vi "Rasnik_20190107.vi"() -> ()   [LabVIEW 2015]
uses:
  GlobalPath.vi
  GlobalData.vi
  <vilib>/Utility/file.llb/Read Delimited Spreadsheet (string).vi
  <vilib>/Utility/file.llb/Write Delimited Spreadsheet (DBL).vi
panel:
  in  "Done?":bool
  in  "Stage":string
  in  "driver off":bool caption="Disconnect the driver from the power supply"
  out "text":string
  out "PanelName":string
  out "appended path":path
  out "Y Diff10":dbl format="%.2f"
  out "Y Diff9":dbl format="%.2f"
  out "Y Diff8":dbl format="%.2f"
  out "Y Diff7":dbl format="%.2f"
  out "Y Diff6":dbl format="%.2f"
  out "Y Diff5":dbl format="%.2f"
  out "Y Diff4":dbl format="%.2f"
  out "Y Diff3":dbl format="%.2f"
  out "Y Diff2":dbl format="%.2f"
  out "Y Diff1":dbl format="%.2f"
  out "X Diff10":dbl format="%.2f"
  out "X Diff9":dbl
  out "X Diff8":dbl format="%.2f"
  out "X Diff7":dbl format="%.2f"
  out "X Diff6":dbl format="%.2f"
  out "X Diff5":dbl format="%.2f"
  out "X Diff4":dbl format="%.2f"
  out "X Diff3":dbl format="%.2f"
  out "X Diff2":dbl format="%.2f"
  out "X Diff1":dbl format="%.2f"
  out "all rows":string[][](array[string])
  out "Y D10":dbl format="%.2f"
  out "Y D9":dbl format="%.2f"
  out "Y D8":dbl format="%.2f"
  out "Y D7":dbl format="%.2f"
  out "Y D6":dbl format="%.2f"
  out "Y D5":dbl format="%.2f"
  out "Y D4":dbl format="%.2f"
  out "Y D3":dbl format="%.2f"
  out "Y D2":dbl format="%.2f"
  out "Y D1":dbl format="%.2f"
  out "X D10":dbl format="%.2f"
  out "X D9":dbl format="%.2f"
  out "X D8":dbl format="%.2f"
  out "X D7":dbl format="%.2f"
  out "X D6":dbl format="%.2f"
  out "X D5":dbl format="%.2f"
  out "X D4":dbl format="%.2f"
  out "X D3":dbl format="%.2f"
  out "X D2":dbl format="%.2f"
  out "X D1":dbl format="%.2f"
  out "y 6":string
  out "y 10":string
  out "y 9":string
  out "y 8":string
  out "y 7":string
  out "y 5":string
  out "y 4":string
  out "y 3":string
  out "y 2":string
  out "y 1":string
  out "x 6":string
  out "x 10":string
  out "x 9":string
  out "x 8":string
  out "x 7":string
  out "x 5":string
  out "x 4":string
  out "x 3":string
  out "x 2":string
  out "x 1":string
  out "output file":path=path "/home/atlas/Micromegas/ProdData/C_CCD/CalcDiscr.txt"
  out "Script":path
  out "Filename selected":path
  out "standard output":string
  in  "Done?":bool
  out "Latest file:":path
  in  "Open Program":bool
  in  "c-ccd 3":bool caption="Setup the electronics for the C-CCD reading:\n- make sure the ethernet cables are connected on the minimal heads\n- check that the cables connecting the driver with the muxs are plugged in\n- CONNECT the driver to the power supply and check that it is connected to the LAN\nIf the measurements show -1 in all c-ccds:\nUNPLUG the driver, WAIT a couple of seconds and REPLUG it"
  in  "c-ccd":bool caption="Read the data file"
  # "Rasmask reading from PCBs on stiffback/table"
  # "Type \"Table\" or \"Stiffback\" for the C-CCDs you want to use:"
  # "Run the C-CCD reading program \n(the 10 Rasmasks are automatically read and the data saved)"
  # "Data file reading"
  # "The most recent data file created by the C-CCD program will be opened.\nOnce the \"read data file\" is clicked, the raw data and displacement should appear on the PCB schematics on the bottom."
  # "Raw Data (mm):"
  # "Calibrated position (mm):"
  # "Difference (wrt Reference reading) (um):"
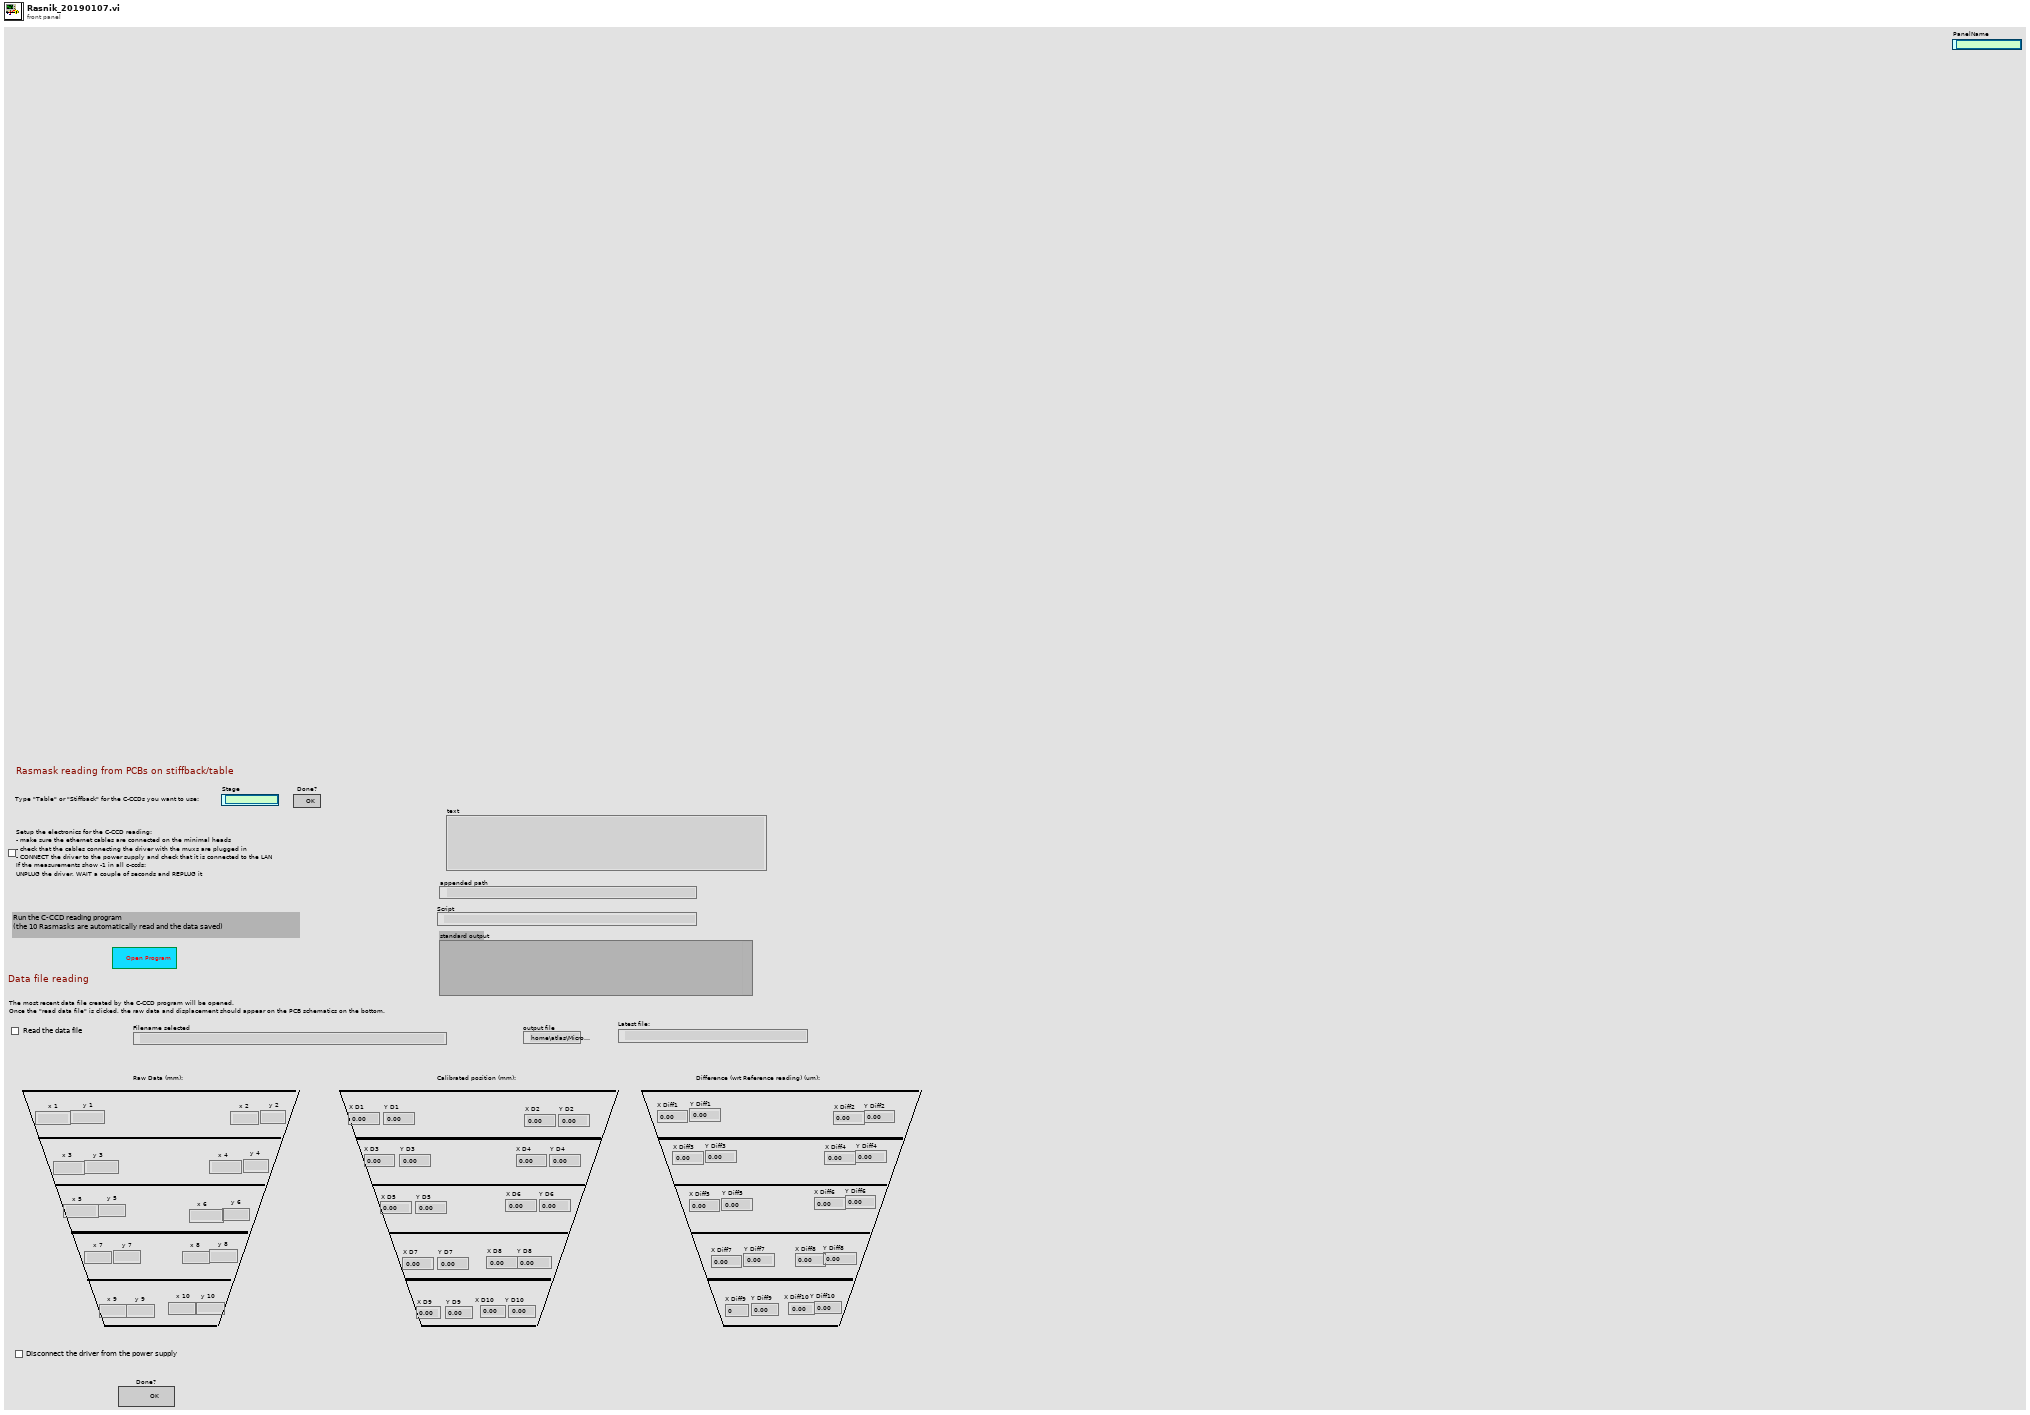
[diagram p1: front panel]
types:
  T1 = enum16{"open", "replace", "create", "open or create", "replace or create", "replace or create with confirmation"}
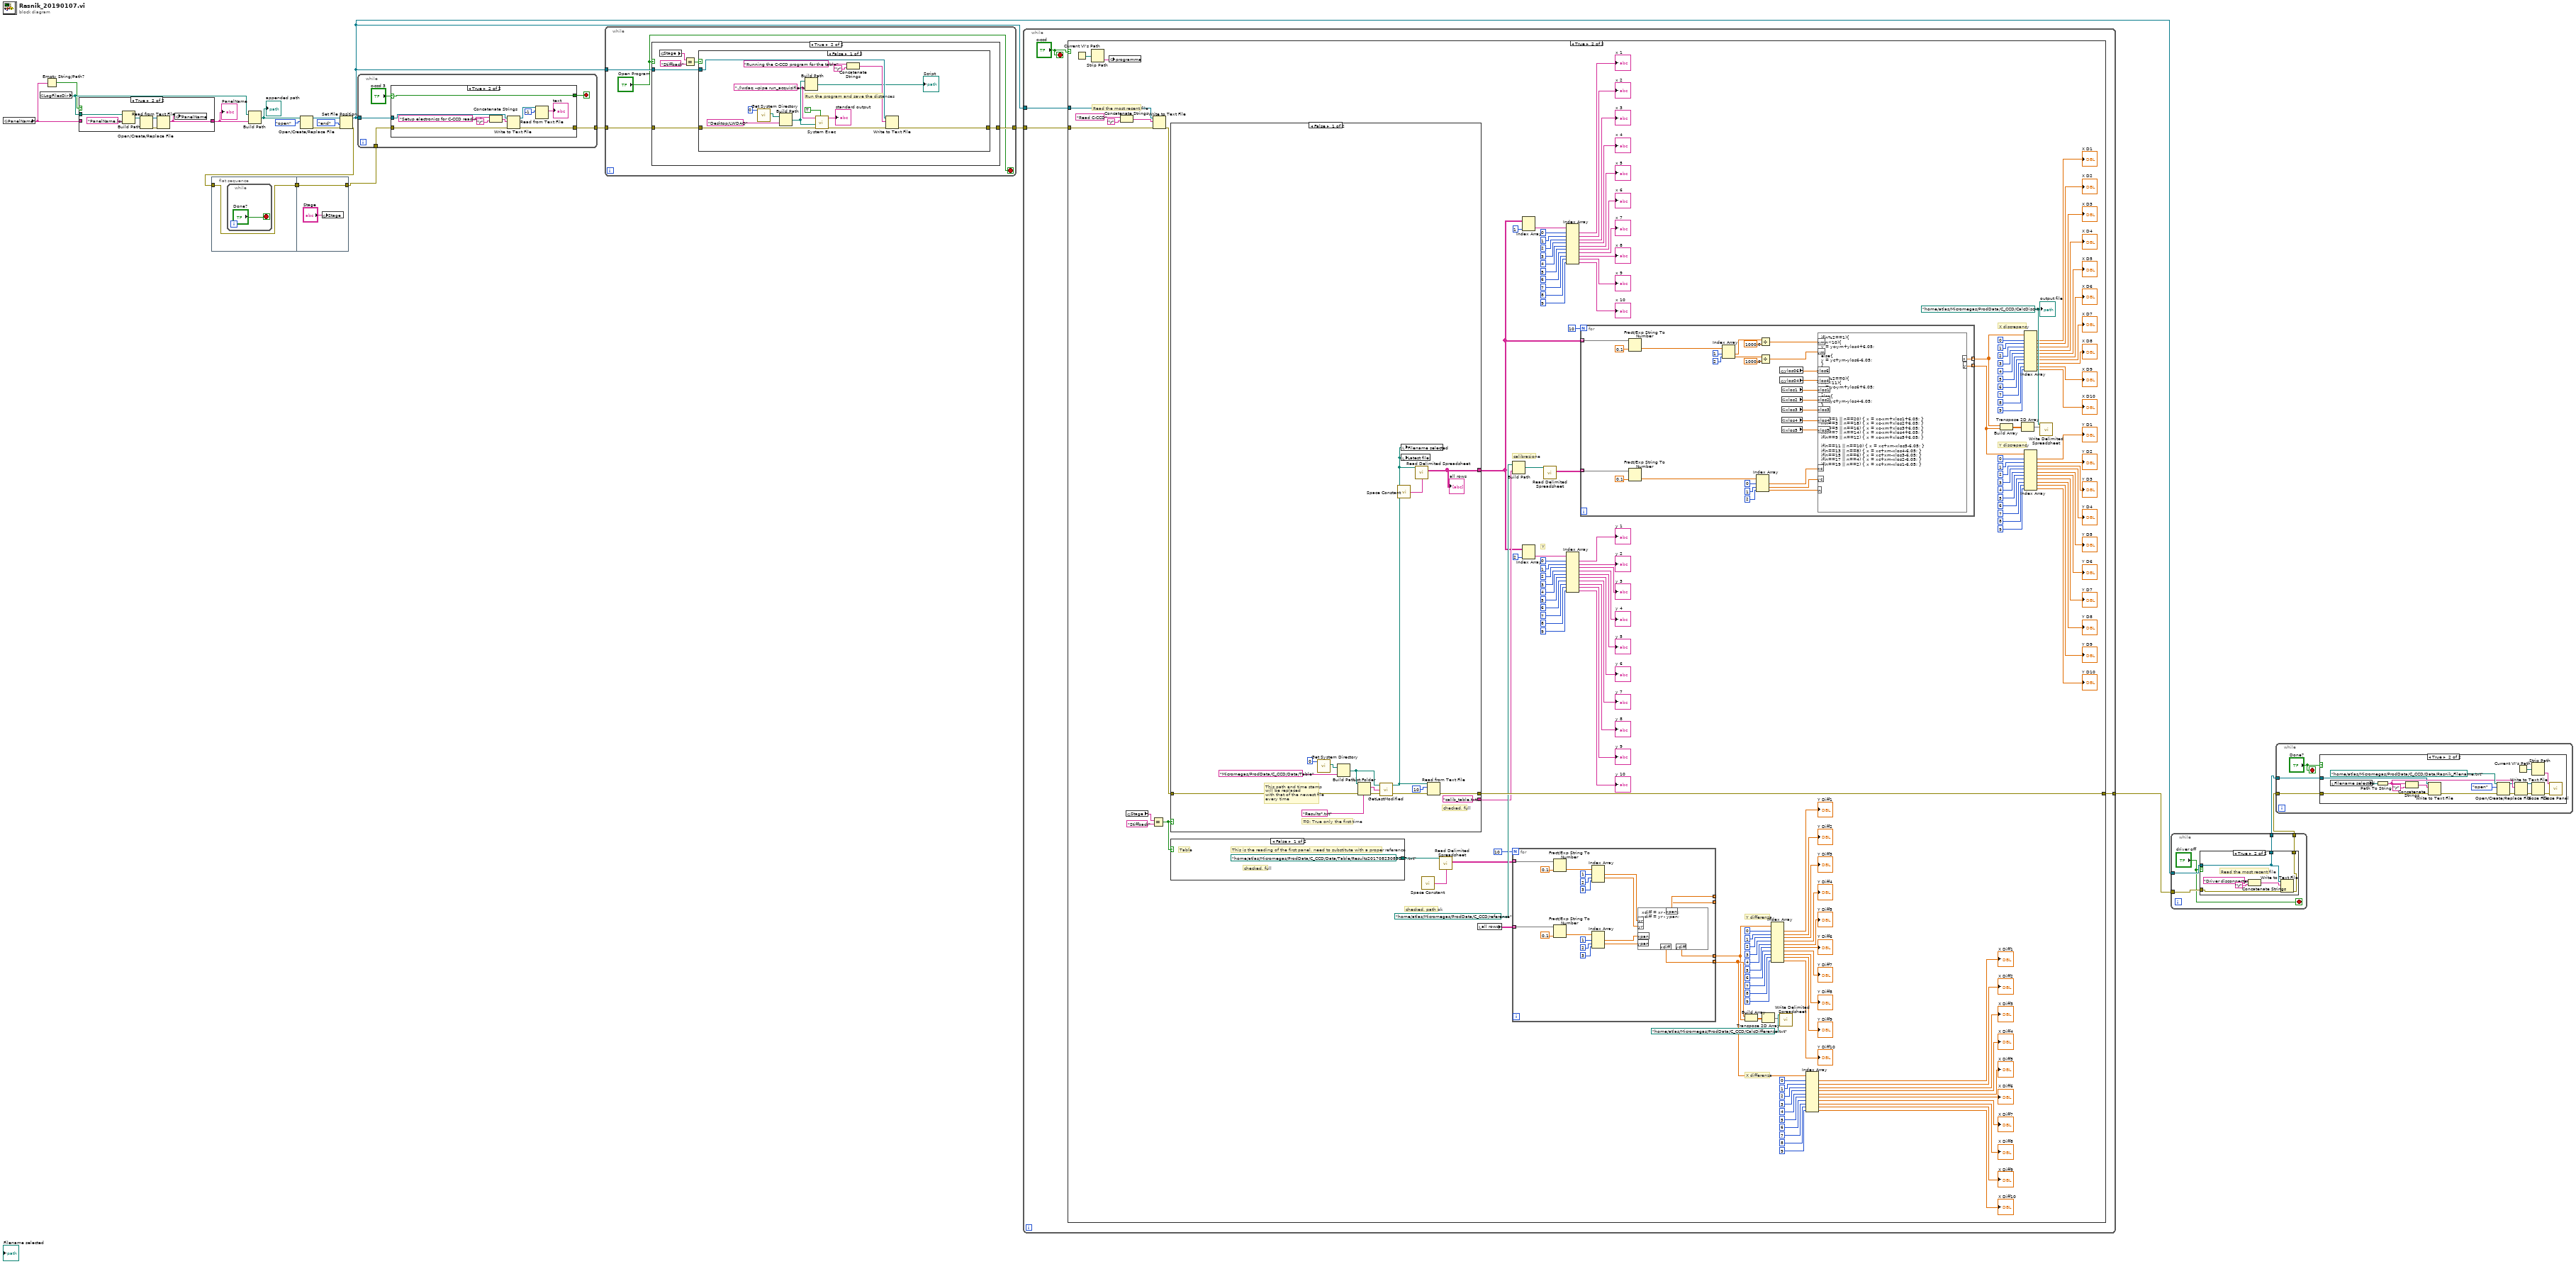
[diagram p0: block diagram]
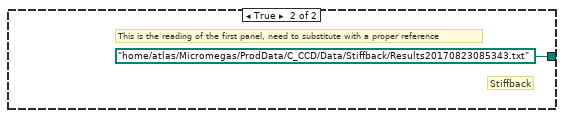
[diagram p5: hidden frame]
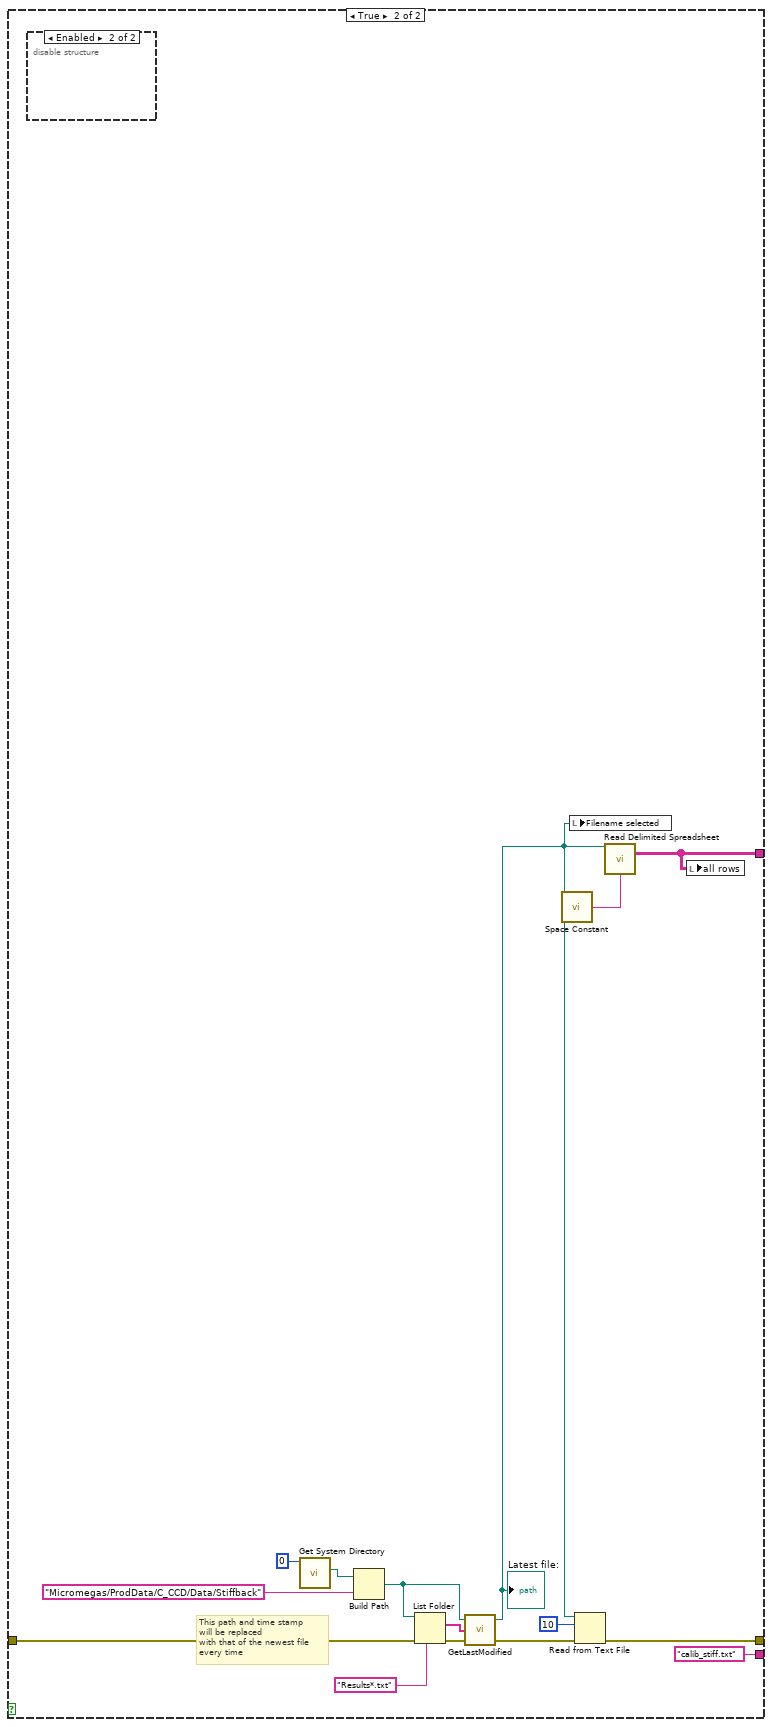
[diagram p6: hidden frame]
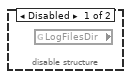
[diagram p7: hidden frame]
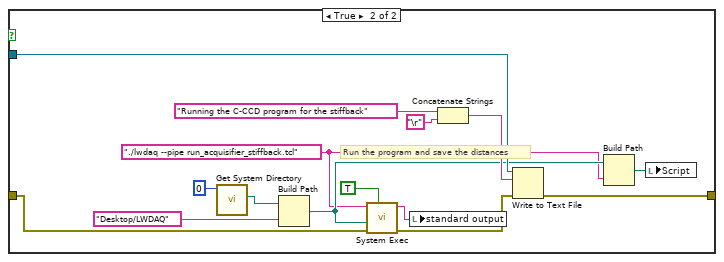
[diagram p10: hidden frame]
diagram:
  n1 = global read "GlobalData.vi" "PanelName"() -> (w14:string)
  n2 = global read "GlobalPath.vi" "LogFilesDir"() -> (w15:path)
  n3 = Empty String/Path?(string/path=w14) -> (empty?=w13:bool)
  n4 = case shown="True" w13 {
    tunnel: w15 -> [_ w25]
    tunnel: [w19 w20] -> w16
    tunnel: w14 -> [w19 _]
    frame False {
    }
    frame True {
      n5 = Build Path(base path=w25, name or relative path="PanelName.log") -> (appended path=w24:path)
      n6 = Open/Create/Replace File(file path (use dialog)=w24) -> (refnum out=w21:refnum<file>, error out=w22:errorcluster)  [unwired: 5 in, 1 out]
      n7 = Read from Text File(file (use dialog)=w21, error in=w22) -> (text=w20:string)  [unwired: 2 in, 3 out]
      n8 = global write "GlobalData.vi" "PanelName"(w20) -> ()
    }
  }
  "PanelName" <- w16
  n9 = flat-sequence {
    tunnel: w3 -> [w26]
    tunnel: [w26] -> w2
    tunnel: [w28] -> w1
    tunnel: w2 -> [w28]
    frame #0 {
      n10 = while {
        stop <- "Done?" stop-if-true
      }
    }
    frame #1 {
      n11 = global write "GlobalData.vi" "Stage"("Stage") -> ()
    }
  }
  n12 = Build Path(base path=w15, name or relative path=w16) -> (appended path=w8:path)
  "appended path" <- w8
  n13 = Open/Create/Replace File(file path (use dialog)=w8, operation (0:open)=T1."open") -> (refnum out=w11:refnum<file>, error out=w12:errorcluster)  [unwired: 4 in, 1 out]
  n14 = Set File Position(refnum=w11, from (0:start)=enum16{"start", "end", "current"}."end", error in=w12) -> (refnum out=w7:refnum<file>, error out=w3:errorcluster)  [unwired: 1 in]
  n15 = while {
    tunnel: w7 -> [w33]
    tunnel: [w31] -> w17
    tunnel: w1 -> [w30]
    stop <- w32 stop-if-true
    n16 = case shown="True" "c-ccd 3" {
      selector: "c-ccd 3" -> [w36 w43]
      tunnel: [w35 w44] -> w31
      tunnel: w33 -> [_ w41]
      tunnel: [w36 w43] -> w32
      tunnel: w30 -> [w35 w42]
      frame False {
      }
      frame True {
        n17 = Concatenate Strings("Setup electronics for C-CCD reading", "\r") -> (w40:string)
        n18 = Write to Text File(file (use dialog)=w41, text=w40, error in=w42) -> (refnum out=w39:refnum<file>, error out=w44:errorcluster)  [unwired: 1 in, 1 out]
        n19 = Read from Text File(file (use dialog)=w39, count=-1) -> (text=→"text":string)  [unwired: 2 in, 3 out]
      }
    }
  }
  n20 = while {
    tunnel: w7 -> [w48]
    tunnel: w17 -> [w50]
    tunnel: [w49] -> w18
    stop <- "Open Program" stop-if-true
    n21 = case shown="True" "Open Program" {
      tunnel: w50 -> [w51 w54]
      tunnel: [w51 w53] -> w49
      tunnel: w48 -> [_ w52]
      frame False {
      }
      frame True {
        n22 = global read "GlobalData.vi" "Stage"() -> (w56:string)
        n23 = Equal?(x=w56, y="Stiffback") -> (x = y?=w55:bool)
        n24 = case shown="False" w55 {
          tunnel: w54 -> [w69 w84]
          tunnel: [w67 w82] -> w53
          tunnel: w52 -> [w66 w81]
          frame False {
            w59 = "./lwdaq --pipe run_acquisifier.tcl"
            # "Run the program and save the distances"
            n25 = call <vilib>:"Get System Directory.vi"("system directory type"=0) -> ("system directory"=w64:path)  [unwired: 10 in]
            n26 = Build Path(base path=w64, name or relative path="Desktop/LWDAQ") -> (appended path=w60:path)
            n27 = Build Path(base path=w60, name or relative path=w59) -> (appended path=→"Script":path)
            n28 = call <vilib>:"System Exec.vi"("wait until completion? (T)"=TRUE, "error in (no error)"=w69, "working directory"=w60, "command line"=w59) -> ("error out"=w68:errorcluster, "standard output"=→"standard output":string)  [unwired: 4 in, 2 out]
            n29 = Concatenate Strings("Running the C-CCD program for the table", "\r") -> (w72:string)
            n30 = Write to Text File(file (use dialog)=w66, text=w72, error in=w68) -> (error out=w67:errorcluster)  [unwired: 1 in, 2 out]
          }
          frame True {
            w75 = "./lwdaq --pipe run_acquisifier_stiffback.tcl"
            # "Run the program and save the distances"
            n31 = call <vilib>:"Get System Directory.vi"("system directory type"=0) -> ("system directory"=w78:path)  [unwired: 10 in]
            n32 = Build Path(base path=w78, name or relative path="Desktop/LWDAQ") -> (appended path=w76:path)
            n33 = call <vilib>:"System Exec.vi"("wait until completion? (T)"=TRUE, "error in (no error)"=w84, "working directory"=w76, "command line"=w75) -> ("error out"=w83:errorcluster, "standard output"=w73:string)  [unwired: 4 in, 2 out]
            n34 = local write "standard output"(w73) -> ()
            n35 = Concatenate Strings("Running the C-CCD program for the stiffback", "\r") -> (w87:string)
            n36 = Write to Text File(file (use dialog)=w81, text=w87, error in=w83) -> (error out=w82:errorcluster)  [unwired: 1 in, 2 out]
            n37 = Build Path(base path=w76, name or relative path=w75) -> (appended path=w74:path)
            n38 = local write "Script"(w74) -> ()
          }
        }
      }
    }
  }
  n39 = while {
    tunnel: w7 -> [w89]
    tunnel: w18 -> [w91]
    tunnel: [w90] -> w6
    stop <- "c-ccd" stop-if-true
    n40 = case shown="True" "c-ccd" {
      tunnel: w91 -> [w92 w242]
      tunnel: [w92 w240] -> w90
      tunnel: w89 -> [_ w239]
      frame False {
      }
      frame True {
        w231 = path "/home/atlas/Micromegas/ProdData/C_CCD/CalcDiscr.txt" ("file path (dialog if empty)")
        # "checked, path ok"
        # "Y differenza"
        # "X differenza"
        # "Y discrepancy"
        # "X discrepancy"
        # "Y"
        # "calibrazione"
        # "Read the most recent file"
        n41 = Current VI's Path() -> (path=w243:path)
        n42 = Strip Path(path=w243) -> (name=w244:string)  [unwired: 1 out]
        n43 = global write "GlobalData.vi" "programma"(w244) -> ()
        n44 = Concatenate Strings("Read C-CCD", "\r") -> (w249:string)
        n45 = global read "GlobalData.vi" "Stage"() -> (w245:string)
        n46 = Equal?(x=w245, y="Stiffback") -> (x = y?=w99:bool)
        n47 = Write to Text File(file (use dialog)=w239, text=w249, error in=w242) -> (error out=w241:errorcluster)  [unwired: 1 in, 2 out]
        n48 = case shown="False" w99 {
          tunnel: w241 -> [w304 w319]
          tunnel: [w314 w329] -> w240
          tunnel: [w302 w316] -> w207
          tunnel: ["calib_table.txt" "calib_stiff.txt"] -> w236
          frame False {
            # "checked, full"
            # "=0: True only the first time"
            # "This path and time stamp\nwill be replaced\nwith that of the newest file \nevery time"
            n49 = call <vilib>:"Get System Directory.vi"("system directory type"=0) -> ("system directory"=w311:path)  [unwired: 10 in]
            n50 = Build Path(base path=w311, name or relative path="Micromegas/ProdData/C_CCD/Data/Table") -> (appended path=w306:path)
            n51 = List Folder(path=w306, pattern="Results*.txt", error in=w304) -> (filenames=w309:string[], error out=w307:errorcluster)  [unwired: 1 in, 2 out]
            n52 = call "GetLastModified.vi"("error in"=w307, "filenames"=w309, "SearchDir"=w306) -> ("error out"=w308:errorcluster, "Path"=w301:path)  [unwired: 1 out]
            n53 = call <vilib>:"Space Constant.vi"() -> ("String"=w303:string)
            n54 = local write "Filename selected"(w301) -> ()
            n55 = local write "Latest file:"(w301) -> ()
            n56 = call-poly <vilib>:"Read Delimited Spreadsheet.vi"("file path (dialog if empty)"=w301, "delimiter (\\t)"=w303) -> ("all rows"=w302:string[][])  [unwired: 8 in, 5 out]
            "all rows" <- w302
            n57 = Read from Text File(file (use dialog)=w301, count=10, error in=w308) -> (error out=w314:errorcluster)  [unwired: 1 in, 3 out]
          }
          frame True {
            # "This path and time stamp\nwill be replaced\nwith that of the newest file \nevery time"
            n58 = disable-structure shown="Enabled" {
              frame Disabled {
                n59 = global read "GlobalPath.vi" "LogFilesDir"() -> ()  [unwired: 1 out]
              }
              frame Enabled {
              }
            }
            n60 = call <vilib>:"Get System Directory.vi"("system directory type"=0) -> ("system directory"=w326:path)  [unwired: 10 in]
            n61 = Build Path(base path=w326, name or relative path="Micromegas/ProdData/C_CCD/Data/Stiffback") -> (appended path=w322:path)
            n62 = List Folder(path=w322, pattern="Results*.txt", error in=w319) -> (filenames=w321:string[], error out=w320:errorcluster)  [unwired: 1 in, 2 out]
            n63 = call "GetLastModified.vi"("error in"=w320, "filenames"=w321, "SearchDir"=w322) -> ("error out"=w323:errorcluster, "Path"=w317:path)  [unwired: 1 out]
            "Latest file:" <- w317
            n64 = call <vilib>:"Space Constant.vi"() -> ("String"=w318:string)
            n65 = local write "Filename selected"(w317) -> ()
            n66 = Read from Text File(file (use dialog)=w317, count=10, error in=w323) -> (error out=w329:errorcluster)  [unwired: 1 in, 3 out]
            n67 = call-poly <vilib>:"Read Delimited Spreadsheet.vi"("file path (dialog if empty)"=w317, "delimiter (\\t)"=w318) -> ("all rows"=w316:string[][])  [unwired: 8 in, 5 out]
            n68 = local write "all rows"(w316) -> ()
          }
        }
        n69 = case shown="False" w99 {
          tunnel: [path "/home/atlas/Micromegas/ProdData/C_CCD/Data/Table/Results20170823085217.txt" ("file path (dialog if empty)") path "/home/atlas/Micromegas/ProdData/C_CCD/Data/Stiffback/Results20170823085343.txt" ("file path (dialog if empty)")] -> w144
          frame False {
            # "checked, full"
            # "This is the reading of the first panel, need to substitute with a proper reference"
            # "Table"
          }
          frame True {
            # "Stiffback"
            # "This is the reading of the first panel, need to substitute with a proper reference"
          }
        }
        n70 = call <vilib>:"Space Constant.vi"() -> ("String"=w96:string)
        n71 = call-poly <vilib>:"Read Delimited Spreadsheet.vi"("file path (dialog if empty)"=w144, "delimiter (\\t)"=w96) -> ("all rows"=w94:string[][])  [unwired: 8 in, 5 out]
        n72 = local read "all rows"() -> (w93:string[][])
        n73 = Build Path(base path=path "/home/atlas/Micromegas/ProdData/C_CCD/reference" ("file path (dialog if empty)"), name or relative path=w236) -> (appended path=w237:path)
        n74 = for {
          N: 10 -> [_]
          tunnel: w94 -> [w269] mode=indexing
          tunnel: w93 -> [w268] mode=indexing
          tunnel: [w257] -> w121 mode=indexing
          tunnel: [w256] -> w100 mode=indexing
          tunnel: [w253] -> _ mode=indexing
          tunnel: [w252] -> _ mode=indexing
          n75 = Fract/Exp String To Number(string=w269, default (0 dbl)=0.1 ("default (0 DBL)")) -> (number=w271:dbl[])  [unwired: 2 in, 1 out]
          n76 = Fract/Exp String To Number(string=w268, default (0 dbl)=0.1 ("default (0 DBL)")) -> (number=w270:dbl[])  [unwired: 2 in, 1 out]
          n77 = Index Array(array=w271, index #1=1, index #2=2, index #3=3) -> (element #1=w261:dbl, element #2=w260:dbl)  [unwired: 1 out]
          n78 = Index Array(array=w270, index #1=1, index #2=2, index #3=3) -> (element #1=w258:dbl, element #2=w259:dbl)  [unwired: 1 out]
          n79 = formula code="xdiff = xr - xpan;\nydiff = yr - ypan;"("xr"=w261, "yr"=w260, "xpan"=w258, "ypan"=w259) -> ("xdiff"=w257:dbl, "ydiff"=w256:dbl, "xr"=w253:dbl, "xpan"=w252:dbl)
        }
        n80 = Index Array(array=w207, index (col)=1 ("disabled index (col)")) -> (element=w229:string[])  [unwired: 1 in]
        n81 = Index Array(array=w207, index (col)=2 ("disabled index (col)")) -> (element=w196:string[])  [unwired: 1 in]
        n82 = call-poly <vilib>:"Read Delimited Spreadsheet.vi"("file path (dialog if empty)"=w237) -> ("all rows"=w235:string[][])  [unwired: 9 in, 5 out]
        n83 = Index Array(array=w229, index #1=0, index #2=1, index #3=2, index #4=3, index #5=4, index #6=5, index #7=6, index #8=7, index #9=8, index #10=9) -> (element #1=→"x 1":string, element #2=→"x 2":string, element #3=→"x 3":string, element #4=→"x 4":string, element #5=→"x 5":string, element #6=→"x 6":string, element #7=→"x 7":string, element #8=→"x 8":string, element #9=→"x 9":string, element #10=→"x 10":string)
        n84 = Index Array(array=w196, index #1=0, index #2=1, index #3=2, index #4=3, index #5=4, index #6=5, index #7=6, index #8=7, index #9=8, index #10=9) -> (element #1=→"y 1":string, element #2=→"y 2":string, element #3=→"y 3":string, element #4=→"y 4":string, element #5=→"y 5":string, element #6=→"y 6":string, element #7=→"y 7":string, element #8=→"y 8":string, element #9=→"y 9":string, element #10=→"y 10":string)
        n85 = for {
          N: 10 -> [_]
          tunnel: w207 -> [w299] mode=indexing
          tunnel: [w298] -> w166 mode=indexing
          tunnel: [w297] -> w145 mode=indexing
          tunnel: w235 -> [w275] mode=indexing
          n86 = Fract/Exp String To Number(string=w299, default (0 dbl)=0.1 ("default (0 DBL)")) -> (number=w294:dbl[])  [unwired: 2 in, 1 out]
          n87 = Fract/Exp String To Number(string=w275, default (0 dbl)=0.1 ("default (0 DBL)")) -> (number=w279:dbl[])  [unwired: 2 in, 1 out]
          n88 = Index Array(array=w294, index #1=1, index #2=2) -> (element #1=w281:dbl, element #2=w285:dbl)
          n89 = Index Array(array=w279, index #1=0, index #2=1, index #3=2) -> (element #1=w274:dbl, element #2=w273:dbl, element #3=w272:dbl)
          n90 = Divide(x=w281, y=1000.0) -> (x/y=w282:dbl)
          n91 = Divide(x=w285, y=1000.0) -> (x/y=w286:dbl)
          n92 = global read "GlobalData.vi" "ylos06"() -> (w288:dbl)
          n93 = global read "GlobalData.vi" "ylos04"() -> (w287:dbl)
          n94 = global read "GlobalData.vi" "xlos1"() -> (w293:dbl)
          n95 = global read "GlobalData.vi" "xlos2"() -> (w292:dbl)
          n96 = global read "GlobalData.vi" "xlos3"() -> (w291:dbl)
          n97 = global read "GlobalData.vi" "xlos4"() -> (w290:dbl)
          n98 = global read "GlobalData.vi" "xlos5"() -> (w289:dbl)
          n99 = formula code="if(n%2==1){\nif(n<10){\ny = yc-ym+ylos4+6.05;\n}\nelse{\ny = yc+ym-ylos6-6.05;\n}\n}\n\nif(n%2==0){\nif(n<11){\ny = yc-ym+ylos6+6.05;\n}\nelse{\ny = yc+ym-ylos4-6.05;\n}\n}\n\nif(n==1 || n==20) { x = xc-xm+xlos1+6.05; } \nif(n==3 || n==18) { x = xc-xm+xlos2+6.05; }\nif(n==5 || n==16) { x = xc-xm+xlos3+6.05; }\nif(n==7 || n==14) { x = xc-xm+xlos4+6.05; }\nif(n==9 || n==12) { x = xc-xm+xlos5+6.05; }\n\nif(n==11 || n==10) { x = xc+xm-xlos5-6.05; } \nif(n==13 || n==8) { x = xc+xm-xlos4-6.05; }\nif(n==15 || n==6) { x = xc+xm-xlos3-6.05; }\nif(n==17 || n==4) { x = xc+xm-xlos2-6.05; }\nif(n==19 || n==2) { x = xc+xm-xlos1-6.05; }"("xm"=w282, "ym"=w286, "ylos6"=w288, "ylos4"=w287, "xlos1"=w293, "xlos2"=w292, "xlos3"=w291, "xlos4"=w290, "xlos5"=w289, "xc"=w274, "yc"=w273, "n"=w272) -> ("x"=w298:dbl, "y"=w297:dbl)
        }
        n100 = Build Array(w121, w100) -> (w97:dbl[][])
        n101 = Transpose 2D Array(2D array=w97) -> (transposed array=w95:dbl[][])
        n102 = Index Array(array=w100, index #1=0, index #2=1, index #3=2, index #4=3, index #5=4, index #6=5, index #7=6, index #8=7, index #9=8, index #10=9) -> (element #1=→"Y Diff1":dbl, element #2=→"Y Diff2":dbl, element #3=→"Y Diff3":dbl, element #4=→"Y Diff4":dbl, element #5=→"Y Diff5":dbl, element #6=→"Y Diff6":dbl, element #7=→"Y Diff7":dbl, element #8=→"Y Diff8":dbl, element #9=→"Y Diff9":dbl, element #10=→"Y Diff10":dbl)
        n103 = call-poly <vilib>:"Write Delimited Spreadsheet.vi"("file path (dialog if empty)"=path "/home/atlas/Micromegas/ProdData/C_CCD/CalcDifferenza.txt", "2D data"=w95) -> ()  [unwired: 12 in, 2 out]
        n104 = Index Array(array=w121, index #1=0, index #2=1, index #3=2, index #4=3, index #5=4, index #6=5, index #7=6, index #8=7, index #9=8, index #10=9) -> (element #1=→"X Diff1":dbl, element #2=→"X Diff2":dbl, element #3=→"X Diff3":dbl, element #4=→"X Diff4":dbl, element #5=→"X Diff5":dbl, element #6=→"X Diff6":dbl, element #7=→"X Diff7":dbl, element #8=→"X Diff8":dbl, element #9=→"X Diff9":dbl, element #10=→"X Diff10":dbl)
        n105 = Build Array(w166, w145) -> (w233:dbl[][])
        n106 = Transpose 2D Array(2D array=w233) -> (transposed array=w232:dbl[][])
        n107 = Index Array(array=w166, index #1=0, index #2=1, index #3=2, index #4=3, index #5=4, index #6=5, index #7=6, index #8=7, index #9=8, index #10=9) -> (element #1=→"X D1":dbl, element #2=→"X D2":dbl, element #3=→"X D3":dbl, element #4=→"X D4":dbl, element #5=→"X D5":dbl, element #6=→"X D6":dbl, element #7=→"X D7":dbl, element #8=→"X D8":dbl, element #9=→"X D9":dbl, element #10=→"X D10":dbl)
        n108 = Index Array(array=w145, index #1=0, index #2=1, index #3=2, index #4=3, index #5=4, index #6=5, index #7=6, index #8=7, index #9=8, index #10=9) -> (element #1=→"Y D1":dbl, element #2=→"Y D2":dbl, element #3=→"Y D3":dbl, element #4=→"Y D4":dbl, element #5=→"Y D5":dbl, element #6=→"Y D6":dbl, element #7=→"Y D7":dbl, element #8=→"Y D8":dbl, element #9=→"Y D9":dbl, element #10=→"Y D10":dbl)
        n109 = call-poly <vilib>:"Write Delimited Spreadsheet.vi"("file path (dialog if empty)"=w231, "2D data"=w232) -> ()  [unwired: 12 in, 2 out]
        "output file" <- w231
      }
    }
  }
  n110 = while {
    tunnel: w7 -> [w335]
    tunnel: w6 -> [w334]
    tunnel: [w333] -> w5
    tunnel: [w332] -> w4
    stop <- "driver off" stop-if-true
    n111 = case shown="True" "driver off" {
      tunnel: w335 -> [w337 w339]
      tunnel: w334 -> [w336 w340]
      tunnel: [w337 w339] -> w333
      tunnel: [w336 w338] -> w332
      frame False {
      }
      frame True {
        # "Read the most recent file"
        n112 = Concatenate Strings("Driver disconnected", "\r") -> (w343:string)
        n113 = Write to Text File(file (use dialog)=w339, text=w343, error in=w340) -> (error out=w338:errorcluster)  [unwired: 1 in, 2 out]
      }
    }
  }
  n114 = while {
    tunnel: w4 -> [w345]
    tunnel: w5 -> [w344]
    stop <- "Done?" stop-if-true
    n115 = case shown="True" "Done?" {
      tunnel: w345 -> [_ w350]
      tunnel: w344 -> [_ w349]
      frame False {
      }
      frame True {
        n116 = local read "Filename selected"() -> (w351:path)
        n117 = Path To String(path=w351) -> (string=w357:string)
        n118 = Concatenate Strings(w357, "\r") -> (w358:string)
        n119 = Write to Text File(file (use dialog)=w349, text=w358, error in=w350) -> (error out=w347:errorcluster)  [unwired: 1 in, 2 out]
        n120 = Open/Create/Replace File(file path (use dialog)=path "/home/atlas/Micromegas/ProdData/C_CCD/Data/Rasnik_Filename.txt", error in=w347, operation (0:open)=T1."open") -> (refnum out=w356:refnum<file>, error out=w353:errorcluster)  [unwired: 3 in, 1 out]
        n121 = Write to Text File(file (use dialog)=w356, text=w357, error in=w353) -> (refnum out=w355:refnum<file>, error out=w354:errorcluster)  [unwired: 1 in, 1 out]
        n122 = Current VI's Path() -> (path=w361:path)
        n123 = Strip Path(path=w361) -> (name=w362:string)  [unwired: 1 out]
        n124 = Close File(refnum=w355, error in=w354) -> (error out=w348:errorcluster)  [unwired: 1 out]
        n125 = call <vilib>:"Close Panel.vi"("error in (no error)"=w348, "VI name"=w362) -> ()  [unwired: 9 in, 1 out]
      }
    }
  }
